vi "Database Logging (parameterized).vi"() -> ()   [LabVIEW 2013]
doc: "This example inserts data into a table named logging in the LabVIEW.mdb database. The data is generated and inserted into the database once per second until you press the Stop button. You can use either of the Playback examples to read the data back into LabVIEW.\n\nThis VI uses a parameterized technique to insert data into the database. Since the SQL query can be parsed once and the data is \"filled in\" when needed, this results in a more efficient VI than the Logging Example. However, the parameterized method is more difficult because it requires you to know more about SQL queries and data types."
uses:
  Auxilliary.llb/DB Tools Parameter Info.ctl
  Auxilliary.llb/DB Tools DataTypes.ctl
  Auxilliary.llb/DB Tools Parameter Dir.ctl
  Auxilliary.llb/DB Tools Column Info.ctl
  Connection.llb/DB Tools Open Connec (Path).vi
  Command.llb/Cmd Delete.vi
  Command.llb/Cmd Set Parameter Value (C).vi
  Command.llb/Cmd Execute.vi
  Recordset.llb/Rec Destroy - Command.vi
  NI_Database_API_64.lvlib
panel:
  in  "column information":T1[](array[typedef])=[{"column name"="RunNumber", "data type"=enum."Long (I32)", "size"=0, "allow null?"=FALSE}, {"column name"="CorePressure", "data type"=enum."Binary", "size"=0, "allow null?"=TRUE}, {"column name"="MaxPressureValue", "data type"=enum."Double (DBL)", "size"=0, "allow null?"=TRUE}, {"column name"="MinPressureValue", "data type"=enum."Double (DBL)", "size"=0, "allow null?"=TRUE}, {"column name"="CoreTemperature", "data type"=enum."Binary", "size"=0, "allow null?"=TRUE}, {"column name"="MaxTemperatureValue", "data type"=enum."Double (DBL)", "size"=0, "allow null?"=TRUE}, {"column name"="MinTemperatureValue", "data type"=enum."Double (DBL)", "size"=0, "allow null?"=TRUE}]
  in  "parameters":T3[](array[typedef])=[{"parameter name"="", "type"=enum."Long (I32)", "direction"=enum."Input", "value"=variant}, {"parameter name"="", "type"=enum."Binary", "direction"=enum."Input", "value"=variant}, {"parameter name"="", "type"=enum."Double (DBL)", "direction"=enum."Input", "value"=variant}, {"parameter name"="", "type"=enum."Double (DBL)", "direction"=enum."Input", "value"=variant}, {"parameter name"="", "type"=enum."Binary", "direction"=enum."Input", "value"=variant}, {"parameter name"="", "type"=enum."Double (DBL)", "direction"=enum."Input", "value"=variant}, {"parameter name"="", "type"=enum."Double (DBL)", "direction"=enum."Input", "value"=variant}]
  out "Number of Records":i32=1
  in  "stop":bool
  out "min temperature value":dbl=296.96037098124657 format="%.2f"
  out "max temperature value":dbl=403.0350221018737 format="%.2f"
  out "min pressure value":dbl=0.29112676548258615 format="%.2f"
  out "max pressure value":dbl=1.56111506192063 format="%.2f"
  out "Core Temperature":dbl[](graph)
  out "Core Pressure":dbl[](graph)
  out "Core Measuments":dbl[][](graph)
  # "INSTRUCTIONS:\n\nRun the VI to insert data into a\ntable called logging in the \nexample database - LabVIEW.mdb.  \nYou can then use the Playback \nVIs to read the data back into \nLabVIEW."
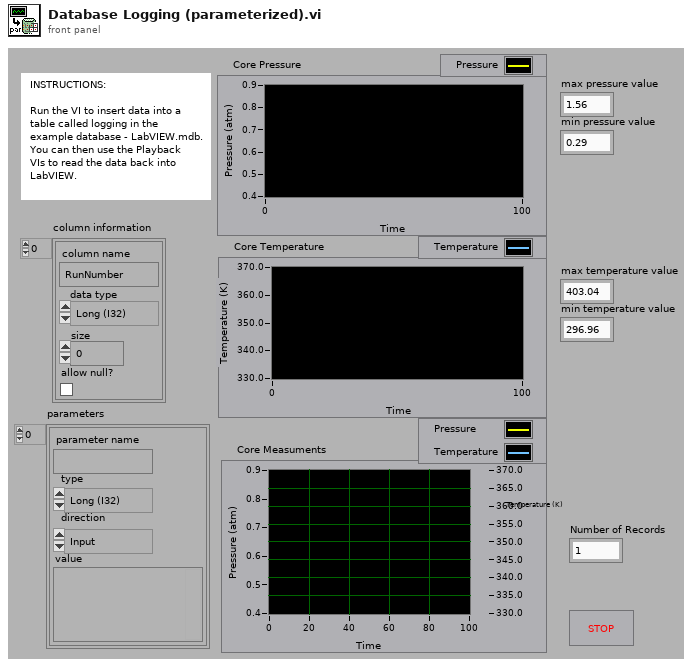
[diagram p1: front panel]
types:
  T1 = typedef "NI_Database_API_64.lvlib/DB Tools Column Info.ctl" = cluster{"column name":string, "data type":T2, "size":i32, "allow null?":bool}
  T2 = typedef "NI_Database_API_64.lvlib/DB Tools DataTypes.ctl" = enum16{"String", "Long (I32)", "Single (SGL)", "Double (DBL)", "Date/Time", "Binary"}
  T3 = typedef "NI_Database_API_64.lvlib/DB Tools Parameter Info.ctl" = cluster{"parameter name":string, "type":T2, "direction":T4, "value":variant}
  T4 = typedef "NI_Database_API_64.lvlib/DB Tools Parameter Dir.ctl" = enum32{"Input", "Output", "Input/Output", "Return Value"}
  T5 = typedef "NI_Database_API_64.lvlib/Conn ObjectReference.ctl" = refnum<k1>
  T6 = typedef "NI_Database_API_64.lvlib/Cmd ObjectReference.ctl" = refnum<k1>
  T7 = typedef "NI_Database_API_64.lvlib/Cmd-Rec Object Reference.ctl" = refnum<k1>
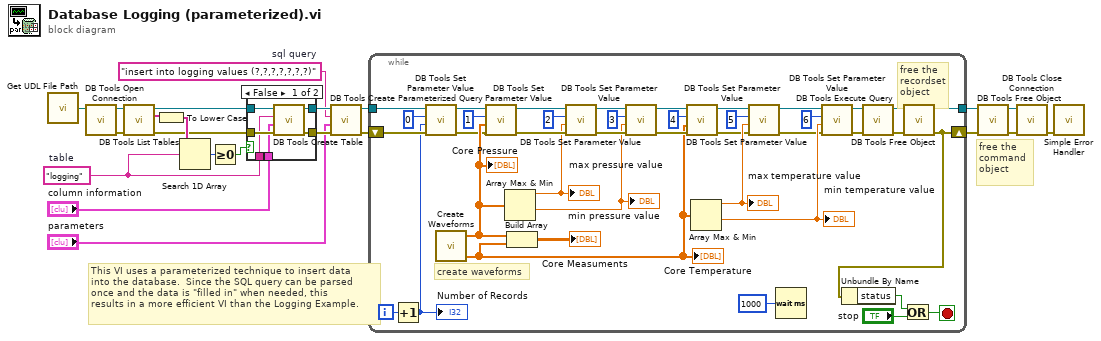
[diagram p0: block diagram]
diagram:
  w20 = "insert into logging values (?,?,?,?,?,?,?)"  # sql query
  w7 = "logging"  # table
  # "free the\ncommand\nobject"
  # "This VI uses a parameterized technique to insert data \ninto the database.  Since the SQL query can be parsed \nonce and the data is \"filled in\" when needed, this \nresults in a more efficient VI than the Logging Example."
  n1 = call "Get UDL File Path.vi"() -> ("UDL file path"=w3:path)  [unwired: 1 in]
  n2 = call-poly "DB Tools Open Connection.vi"("connection information"=w3) -> ("error out"=w13:errorcluster, "connection reference"=w12:T5)  [unwired: 7 in]
  n3 = call "DB Tools List Tables.vi"("error in (no error)"=w13, "connection reference"=w12) -> ("error out"=w6:errorcluster, "tables"=w10:string[], "connection reference out"=w5:T5)  [unwired: 3 in]
  n4 = To Lower Case(string=w10) -> (all lower case string=w11:string[])
  n5 = Search 1D Array(1D array=w11, element=w7) -> (index of element=w8:i32)  [unwired: 1 in]
  n6 = Greater Or Equal To 0?(x=w8) -> (x >= 0?=w9:bool)
  n7 = case shown="False" w9 {
    tunnel: w5 -> [w27 w30]
    tunnel: w6 -> [w28 w29]
    tunnel: [w26 w30] -> w21
    tunnel: [w25 w29] -> w22
    tunnel: w7 -> [w24 _]
    tunnel: "column information" -> [w23 _]
    frame False {
      n8 = call "DB Tools Create Table.vi"("error in (no error)"=w28, "column information"=w23, "table"=w24, "connection reference"=w27) -> ("error out"=w25:errorcluster, "connection reference out"=w26:T5)  [unwired: 4 in]
    }
    frame True {
    }
  }
  n9 = call "DB Tools Create Parameterized Query.vi"("error in (no error)"=w22, "parameters"="parameters", "SQL query"=w20, "connection reference"=w21) -> ("error out"=w15:errorcluster, "command reference"=w18:T6)  [unwired: 3 in, 1 out]
  n10 = while {
    tunnel: w18 -> [w38]
    shift-right: [w52] -> w17
    shift-left: w15 -> [w37]
    tunnel: [w31] -> w1
    i -> [w67]
    stop <- w64 stop-if-true
    # "free the\nrecordset\nobject"
    # "create waveforms"
    n11 = Increment(x=w67) -> (x+1=w34:i32)
    "Number of Records" <- w34
    n12 = call-poly "DB Tools Set Parameter Value.vi"("error in (no error)"=w37, "value"=w34, "parameter index"=0, "command reference"=w38) -> ("error out"=w36:errorcluster, "command reference out"=w35:T6)  [unwired: 4 in]
    n13 = call "Create Waveforms.vi"() -> ("core pressure"=w43:dbl[], "core temperature"=w42:dbl[])  [unwired: 3 in]
    "Core Pressure" <- w43
    "Core Temperature" <- w42
    n14 = call-poly "DB Tools Set Parameter Value.vi"("error in (no error)"=w36, "value"=w43, "parameter index"=1, "command reference"=w35) -> ("error out"=w62:errorcluster, "command reference out"=w61:T6)  [unwired: 4 in]
    n15 = Array Max & Min(array=w43) -> (max value=w41:dbl, min value=w45:dbl)  [unwired: 2 out]
    "max pressure value" <- w41
    "min pressure value" <- w45
    n16 = Build Array(w43, w42) -> (→"Core Measuments":dbl[][])
    n17 = call-poly "DB Tools Set Parameter Value.vi"("error in (no error)"=w62, "value"=w41, "parameter index"=2, "command reference"=w61) -> ("error out"=w60:errorcluster, "command reference out"=w39:T6)  [unwired: 4 in]
    n18 = call-poly "DB Tools Set Parameter Value.vi"("error in (no error)"=w60, "value"=w45, "parameter index"=3, "command reference"=w39) -> ("error out"=w59:errorcluster, "command reference out"=w33:T6)  [unwired: 4 in]
    n19 = call-poly "DB Tools Set Parameter Value.vi"("error in (no error)"=w59, "value"=w42, "parameter index"=4, "command reference"=w33) -> ("error out"=w58:errorcluster, "command reference out"=w57:T6)  [unwired: 4 in]
    n20 = Array Max & Min(array=w42) -> (max value=w68:dbl, min value=w70:dbl)  [unwired: 2 out]
    "max temperature value" <- w68
    "min temperature value" <- w70
    n21 = call-poly "DB Tools Set Parameter Value.vi"("error in (no error)"=w58, "value"=w68, "parameter index"=5, "command reference"=w57) -> ("error out"=w55:errorcluster, "command reference out"=w56:T6)  [unwired: 4 in]
    n22 = Wait (ms)(milliseconds to wait=u32 1000) -> ()  [unwired: 1 out]
    n23 = call-poly "DB Tools Set Parameter Value.vi"("error in (no error)"=w55, "value"=w70, "parameter index"=6, "command reference"=w56) -> ("error out"=w32:errorcluster, "command reference out"=w44:T6)  [unwired: 4 in]
    n24 = call-poly "DB Tools Execute Query.vi"("error in (no error)"=w32, "command reference"=w44) -> ("error out"=w54:errorcluster, "command-recordset reference"=w53:T7)  [unwired: 6 in]
    n25 = call-poly "DB Tools Free Object.vi"("error in (no error)"=w54, "command-recordset reference"=w53) -> ("error out"=w52:errorcluster, "command reference"=w31:T6)  [unwired: 8 in]
    n26 = Unbundle By Name(w52) -> ("status"=w66:bool)
    n27 = Or(x=w66, y="stop") -> (x .or. y?=w64:bool)
  }
  n28 = call-poly "DB Tools Free Object.vi"("error in (no error)"=w17, "command reference"=w1) -> ("error out"=w16:errorcluster, "connection reference"=w2:T5)  [unwired: 8 in]
  n29 = call "DB Tools Close Connection.vi"("error in (no error)"=w16, "connection reference"=w2) -> ("error out"=w14:errorcluster)  [unwired: 5 in]
  n30 = call <vilib>:"Simple Error Handler.vi"("error in (no error)"=w14) -> ()  [unwired: 4 in, 5 out]
